vi "RxTestExample.vi"() -> ()   [LabVIEW 2015]
uses:
  PhyPort.ctl
  BW.ctl
  VISAOperation.ctl
  ONOFF.ctl
panel:
  out "ON/OFFCMD":string="SOUR:RFSG:GPRF:STAT ON"
  out "GenerationConfigCMD":string[](array[string])=["SOURce:RFSG:WLAN:NCHains 1", "SOURce:RFSG:WLAN:CSEGment1:PORTname 'Port0'", "SOURce:RFSG:WLAN:CSEGment2:PORTname 'Port5'", "SOURce:RFSG:WLAN:CSEGment1:FREQuency:CENTer 5180000000.000000", "SOURce:RFSG:WLAN:CSEGment2:FREQuency:CENTer 5700000000.000000", "SOURce:RFSG:WLAN:CSEGment1:POWer:LEVel -30", "SOURce:RFSG:WLAN:CSEGment2:POWer:LEVel -30", "SOURce:RFSG:WLAN:ACTive:ALL:ENABle 1", "SOURce:RFSG:WLAN:CSEGment1:EATTenuation 0", "SOURce:RFSG:WLAN:CSEGment2:EATTenuation 0", "SOURce:RFSG:WLAN:PACKet:MCSindex 9", "SOURce:RFSG:WLAN:PACKet:NSTS 1", "SOURce:RFSG:WLAN:BWIDth 80+80", "SOURce:RFSG:WLAN:IDLEtime 0.001000", "SOURce:RFSG:WLAN:PHY VHT", "SOURce:RFSG:WLAN:PACKet:GINTerval LONG", "SOURce:RFSG:WLAN:PACKet:COUNt -1", "SOURce:RFSG:WLAN:PACKet:PAYLoad:FECType BCC", "SOURce:RFSG:WLAN:PACKet:PAYLoad:MAC 'FF:FF:FF:FF:FF:FF'", "SOURce:RFSG:WLAN:PACKet:PAYLoad:LENGth 1500", "*wai"]
  in  "GenerationConfig":T3={"ExternalAtt"=0.0, "Freq"=5180000000.0, "RxPwr"=-30.0, "PacketNumber"=100, "WaveformName(WithType)"="ac80mcs9.tdms", "PhyPort"=enum."Port0", "PhyPort2"=enum."Port5", "Freq2"=5700000000.0, "BW"=enum."80P80M", "MCSIndex"=9.0} {"Freq2" format="%#_13g"; "RxPwr" format="%#_13g"; "Freq" format="%#_13g"; "ExternalAtt" format="%#_13g"}
  in  "VISA resource name":refnum<visa-resource-name>="TCPIP0::10.144.41.54::inst0::INSTR"
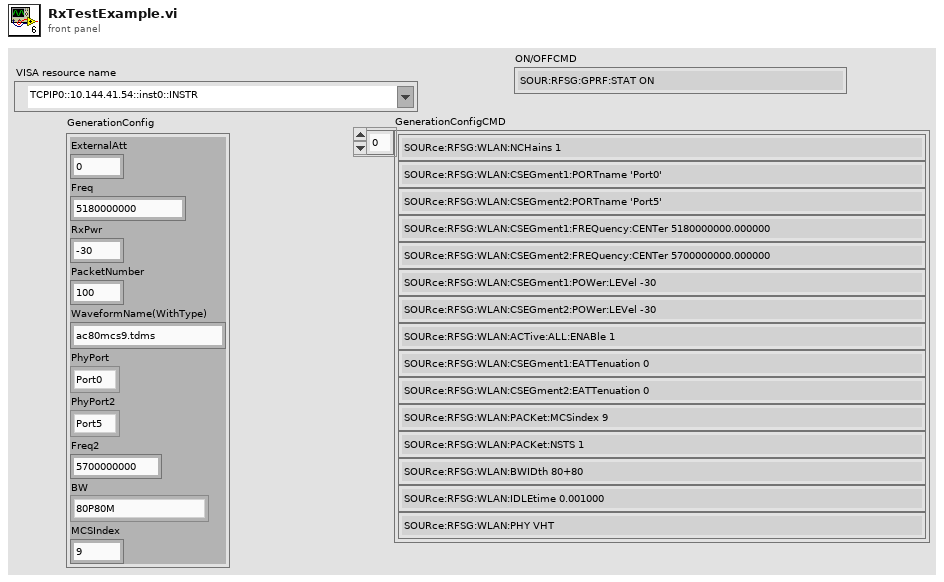
[diagram p1: front panel]
types:
  T1 = typedef "PhyPort.ctl" = enum16{"Port0", "Port1", "Port2", "Port3", "Port4", "Port5", "Port6", "Port7"}
  T2 = typedef "BW.ctl" = enum16{"5M", "10M", "20M", "40M", "80M", "80P80M", "160M"}
  T3 = cluster{"ExternalAtt":dbl, "Freq":dbl, "RxPwr":dbl, "PacketNumber":i32, "WaveformName(WithType)":string, "PhyPort":T1, "PhyPort2":T1, "Freq2":dbl, "BW":T2, "MCSIndex":dbl}
  T4 = typedef "ONOFF.ctl" = u16
  T5 = typedef "VISAOperation.ctl" = enum16{"RunFile", "OpenDebugPanel", "ReadError", "ReadSTB", "Reset", "Clean", "CloseVISA", "RunCMD", "OpenVISA"}
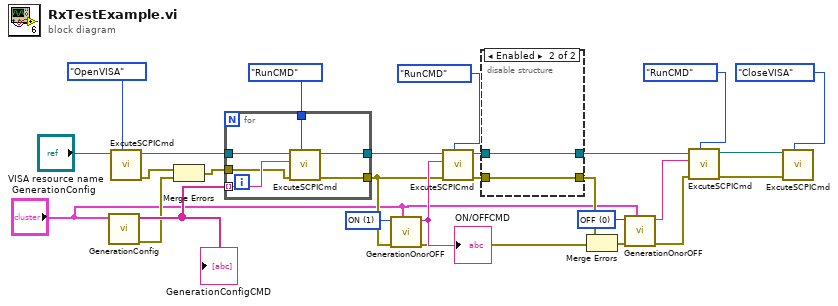
[diagram p0: block diagram]
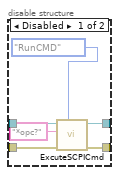
[diagram p2: hidden frame]
diagram:
  w7 = T4 0 items=["OFF", "ON"] ("ON/OFF")
  w8 = T4 1 items=["OFF", "ON"] ("ON/OFF")
  n1 = call "GenerationConfig.vi"("GenerationConfig"="GenerationConfig") -> ("error out"=w15:errorcluster, "GenerationConfigCMD"=w23:string[])  [unwired: 9 in]
  "GenerationConfigCMD" <- w23
  n2 = call "ExcuteSCPICmd.vi"("VISAOperation"=VISAOperation."OpenVISA", "VISA resource name"="VISA resource name") -> ("error out"=w16:errorcluster, "reference out"=w25:refnum<visa-resource-name>)  [unwired: 6 in, 2 out]
  n3 = Merge Errors(w16, w15) -> (w14:errorcluster)
  n4 = for {
    tunnel: w25 -> [w33]
    tunnel: VISAOperation."RunCMD" ("VISAOperation") -> [w32]
    tunnel: w23 -> [w31] mode=indexing
    tunnel: [w30] -> w22
    tunnel: w14 -> [w29]
    tunnel: [w28] -> w13
    n5 = call "ExcuteSCPICmd.vi"("VISAOperation"=w32, "error in (no error)"=w29, "Run Command"=w31, "VISA resource name"=w33) -> ("error out"=w28:errorcluster, "reference out"=w30:refnum<visa-resource-name>)  [unwired: 4 in, 2 out]
  }
  n6 = call "GenerationOnorOFF.vi"("GenerationConfig"="GenerationConfig", "error in (no error)"=w13, "ON/OFF"=w8) -> ("error out"=w11:errorcluster, "ON/OFFCMD"=w20:string)  [unwired: 7 in]
  "ON/OFFCMD" <- w20
  n7 = call "ExcuteSCPICmd.vi"("VISAOperation"=VISAOperation."RunCMD", "error in (no error)"=w13, "Run Command"=w20, "VISA resource name"=w22) -> ("error out"=w6:errorcluster, "reference out"=w4:refnum<visa-resource-name>)  [unwired: 4 in, 2 out]
  n8 = disable-structure shown="Enabled" {
    disable-tunnel: w6 -> [w39 w40]
    disable-tunnel: [w38 w40] -> w5
    disable-tunnel: w4 -> [w37 w41]
    disable-tunnel: [w36 w41] -> w3
    frame Disabled {
      n9 = call "ExcuteSCPICmd.vi"("VISAOperation"=VISAOperation."RunCMD", "error in (no error)"=w39, "Run Command"="*opc?", "VISA resource name"=w37) -> ("error out"=w38:errorcluster, "reference out"=w36:refnum<visa-resource-name>)  [unwired: 4 in, 2 out]
    }
    frame Enabled {
    }
  }
  n10 = Merge Errors(w5, w11) -> (w12:errorcluster)
  n11 = call "GenerationOnorOFF.vi"("GenerationConfig"="GenerationConfig", "error in (no error)"=w12, "ON/OFF"=w7) -> ("error out"=w10:errorcluster, "ON/OFFCMD"=w18:string)  [unwired: 7 in]
  n12 = call "ExcuteSCPICmd.vi"("VISAOperation"=VISAOperation."RunCMD", "error in (no error)"=w10, "Run Command"=w18, "VISA resource name"=w3) -> ("error out"=w9:errorcluster, "reference out"=w2:refnum<visa-resource-name>)  [unwired: 4 in, 2 out]
  n13 = call "ExcuteSCPICmd.vi"("VISAOperation"=VISAOperation."CloseVISA", "error in (no error)"=w9, "VISA resource name"=w2) -> ()  [unwired: 5 in, 4 out]
